vi "CSM-FileSyncWindow.vi"(7 "Name(FileSync)":string="FileSync") -> ()   [LabVIEW 2020, in "CSM-FileSync.lvlib"]
doc: "------------- lvcsm -------------\n[CSMStates]\nItem 0 = \"Event Structure\"\nItem 1 = \"Idle\"\nItem 2 = \"CSM Documentation\"\nItem 3 = \"VI Reference\"\nItem 4 = \"Error Handler\"\nItem 5 = \"Critical Error\"\nItem 6 = \"Target Timeout Error\"\nItem 7 = \"Target Error\"\nItem 8 = \"Async Response\"\nItem 9 = \"Response\"\nItem 10 = \"Async Message Posted\"\nItem 11 = \"Initialize Core Data\"\nItem 12 = \"Exit\"\nItem 13 = \"Data: Initialize\"\nItem 14 = \"Data: Cleanup\"\nItem 15 = \"Events: Register\"\nItem 16 = \"Events: Unregister\"\nItem 17 = \"UI: Initialize\"\nItem 18 = \"UI: Cursor Set\"\nItem 19 = \"UI: Front Panel State\"\nItem 20 = \"Macro: Initialize\"\nItem 21 = \"Macro: Exit\"\nItem 22 = \"API: Update List\"\nItem 23 = \"API: Update Connected Status\"\nItem 24 = \"API: Update Statusbar\"\nItem 25 = \"API: Link to Sync Engine\"\n\n[CSMStatus]\nItem 0 = \"Error Occurred@Error Handler\""
uses:
  CSM-FileSync.lvlib
  6641ad17-a0ad-4bac-bb5f-2ef3ab68202a.vi
  8cb7b144-fc6f-4ba1-ba8b-99306a1222b8.vi
  fb79005b-40a1-4b02-92b0-90b422e2c596.vi
  <userlib>/_NEVSTOP/Communicable State Machine(CSM)/AdvanceAPI/CSM - Revert Arguments-Safe String.vi
  <userlib>/_NEVSTOP/Communicable State Machine(CSM)/_Shared/Trim Single-line Text.vi
  <userlib>/_NEVSTOP/Communicable State Machine(CSM)/AdvanceAPI/CSM - Make String Arguments Safe.vi
  <userlib>/_NEVSTOP/Communicable State Machine(CSM)/AdvanceAPI/CSM - Break Down Multiple States String.vi
  <userlib>/_NEVSTOP/Communicable State Machine(CSM)/AdvanceAPI/CSM - Compact Multiple States.vi
  <userlib>/_NEVSTOP/Communicable State Machine(CSM)/AdvanceAPI/CSM - Keywords.vi
  <userlib>/_NEVSTOP/Communicable State Machine(CSM)/addons/MassData-Parameter/_support/FGV-MassData(lvlibp).vi
  <userlib>/_NEVSTOP/Communicable State Machine(CSM)/addons/API-String-Arugments-Support/_Support/Convert API String Arguments to Data(variant).vi
  <userlib>/_NEVSTOP/Communicable State Machine(CSM)/_Polymophic/CSM - Replace Marks in Messages.vi
  <userlib>/_NEVSTOP/Communicable State Machine(CSM)/Communicable State Machine.lvlib
panel:
  in  "Status":i32[](listbox)
  out "Statusbar":string
  out "Connected":bool
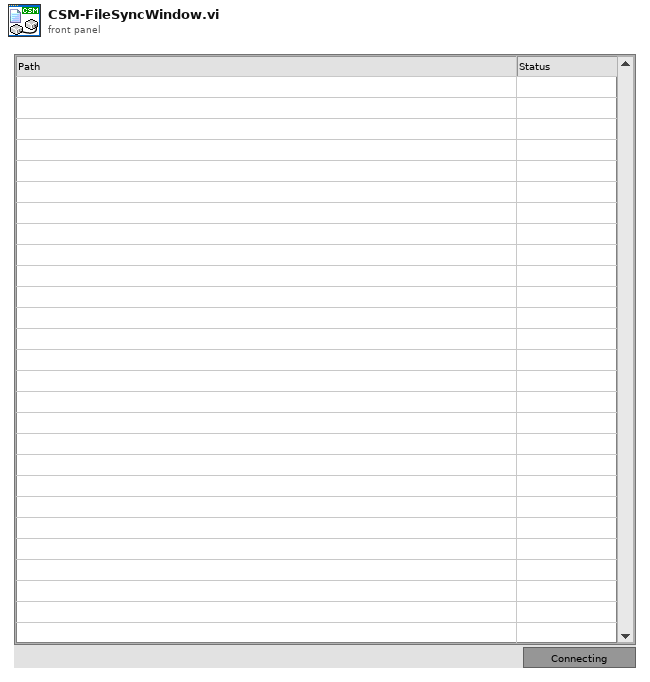
[diagram p1: front panel]
types:
  T1 = enum32{"Invalid", "Standard", "Closed", "Hidden", "Minimized", "Maximized"}
  T2 = enum32{"invalid app kind", "Development System", "Run Time System", "Student Edition", "Embedded LabVIEW", "Evaluation", "Custom"}
  T3 = cluster{"Upload List":path[], "UploadingFile":path}
  T4 = typedef "Communicable State Machine.lvlib/_CSM_Response Source Message.ctl" = cluster{"‘State":string, "’Arguments":string, "’Error":errorcluster}
  T5 = cluster{"Current VI Reference":refnum<vi>, "Close Panel on Exit?":bool}
  T6 = cluster{"Core":cluster{"Current VI Reference":refnum<vi>, "Close Panel on Exit?":bool}, "Status":refnum<vi>}
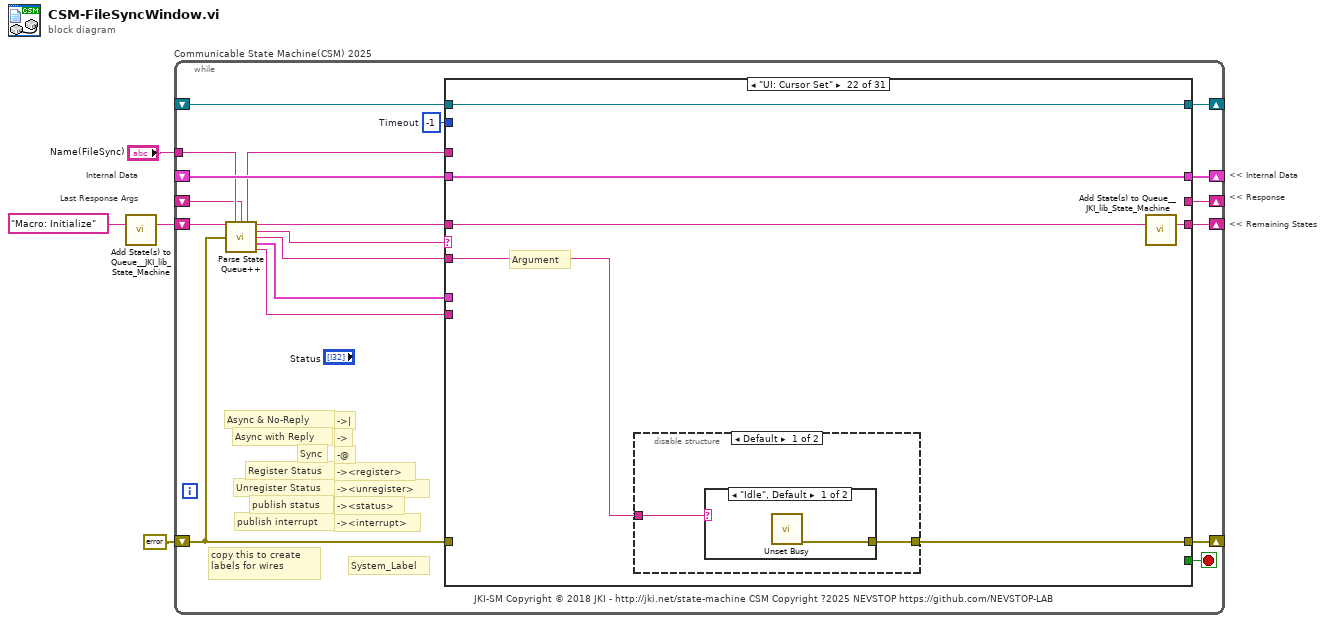
[diagram p0: block diagram]
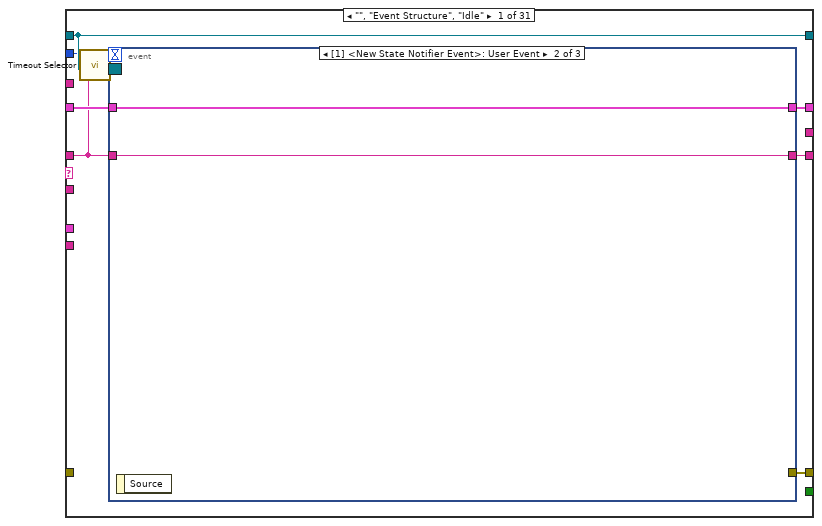
[diagram p2: hidden frame]
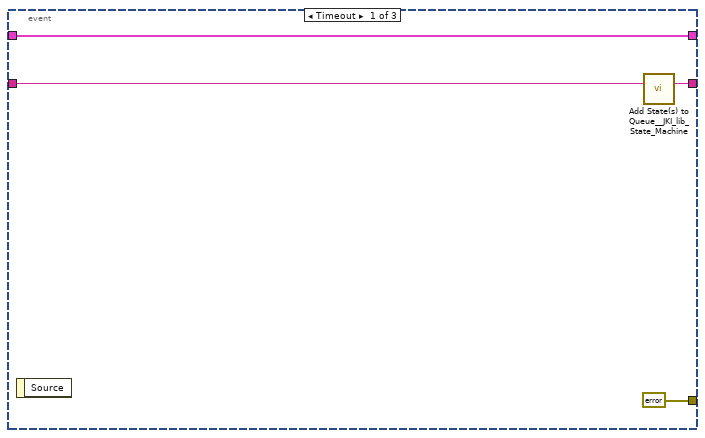
[diagram p3: hidden frame]
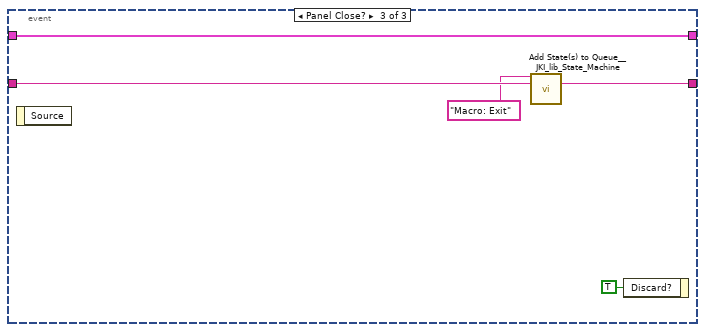
[diagram p4: hidden frame]
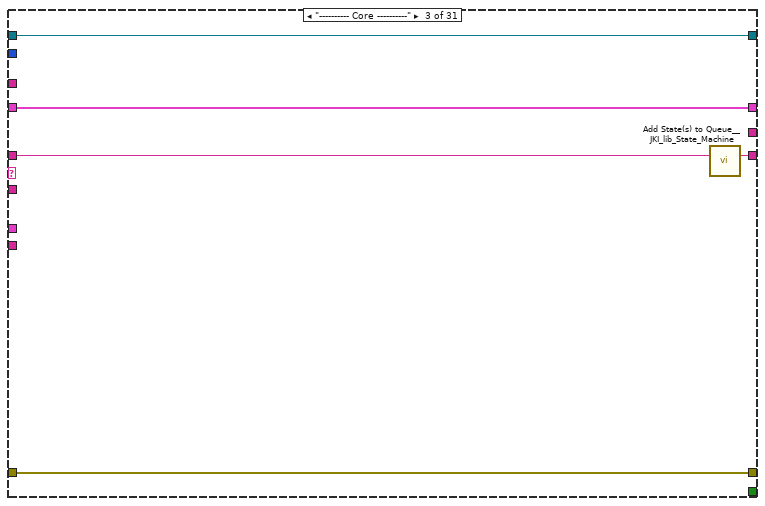
[diagram p6: hidden frame]
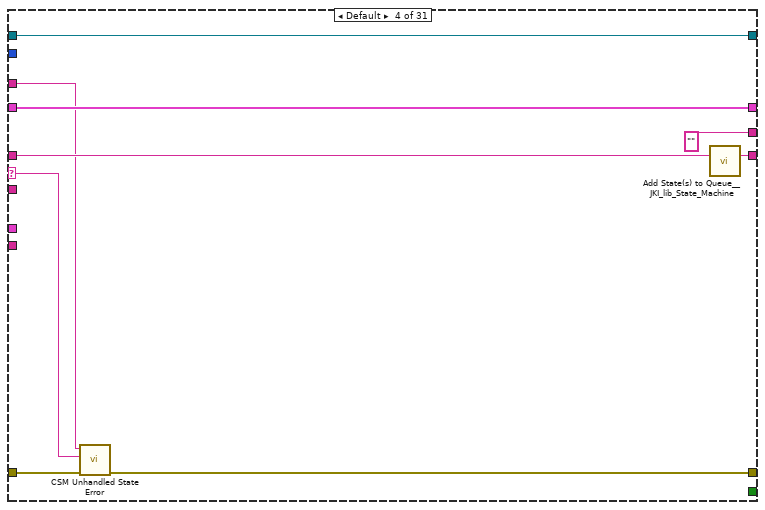
[diagram p7: hidden frame]
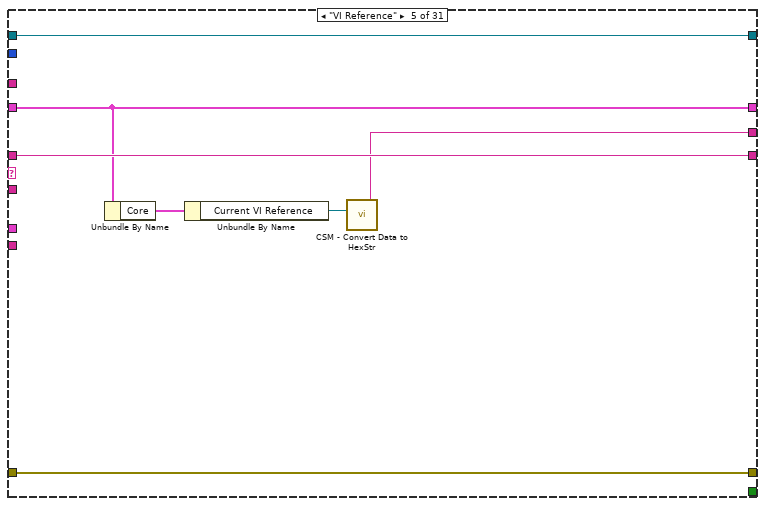
[diagram p8: hidden frame]
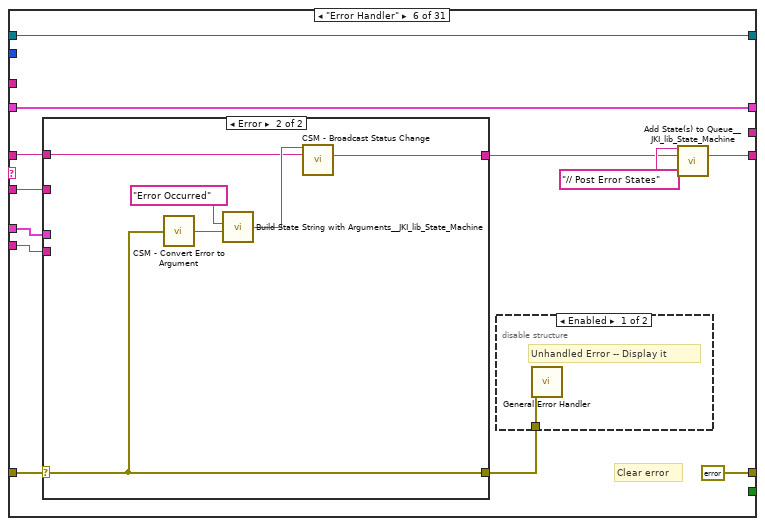
[diagram p9: hidden frame]
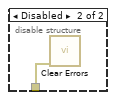
[diagram p10: hidden frame]
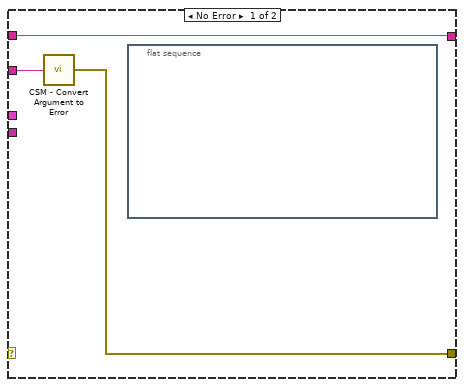
[diagram p11: hidden frame]
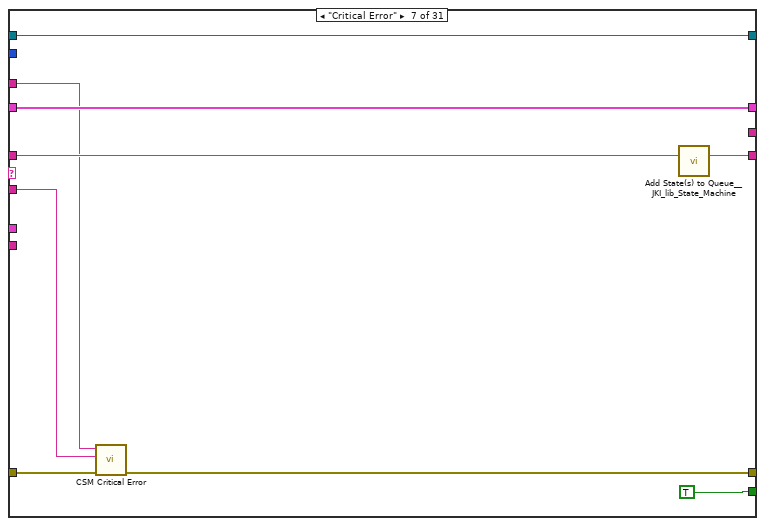
[diagram p12: hidden frame]
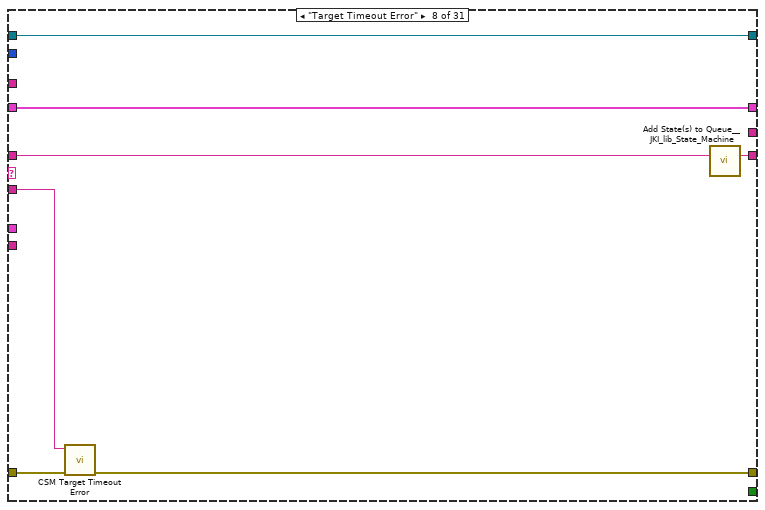
[diagram p13: hidden frame]
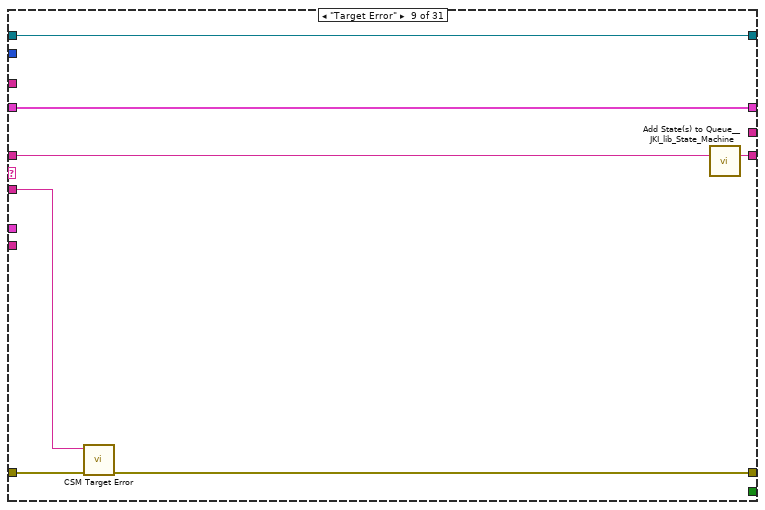
[diagram p14: hidden frame]
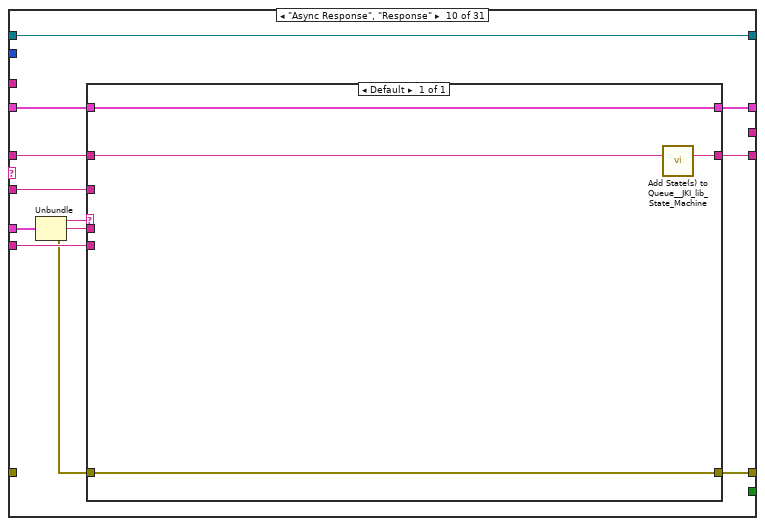
[diagram p15: hidden frame]
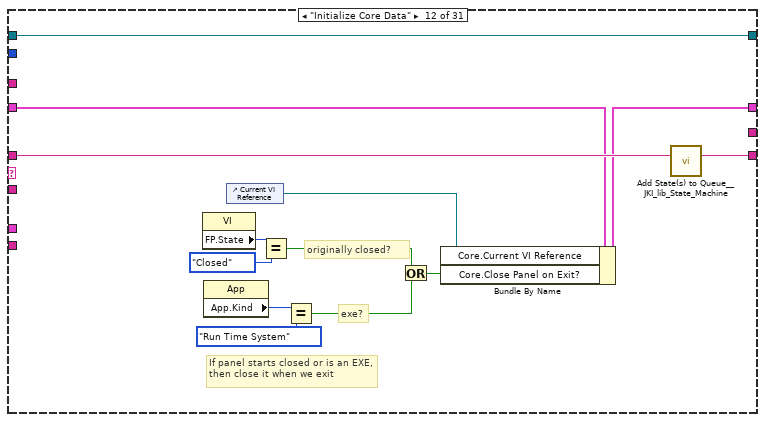
[diagram p17: hidden frame]
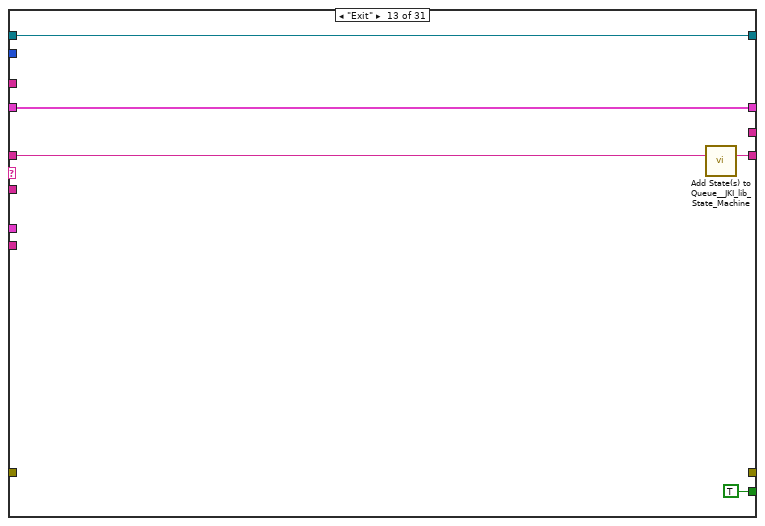
[diagram p18: hidden frame]
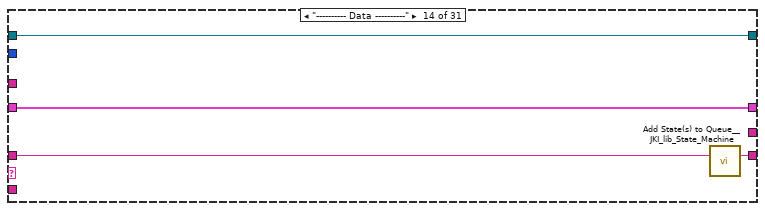
[diagram p19: hidden frame]
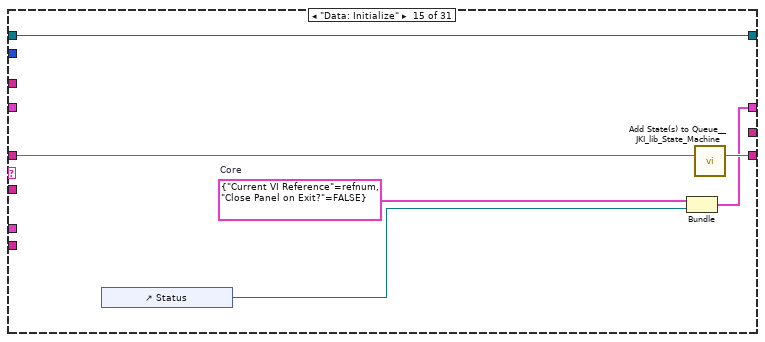
[diagram p20: hidden frame]
diagram:
  # "Last Response Args"
  # "Internal Data"
  # "<< Internal Data"
  # "<< Response"
  # "<< Remaining States"
  n1 = call <vilib>:"Add State(s) to Queue__JKI_lib_State_Machine.vi"("State(s) in (\"\")"="Macro: Initialize" ("Init State(\"Macro: Initialize\")")) -> ("States Out"=w3:string)  [unwired: 14 in]
  n2 = while "Communicable State Machine(CSM) 2025" {
    shift-right: [w18] -> _
    shift-left: _ -> [w17]
    shift-right: [w21] -> _
    shift-left: errorcluster {"status"=FALSE, "code"=0, "source"=""} ("error in") -> [w15]
    shift-right: [w20] -> _
    shift-left: w3 -> [w22]
    tunnel: "Name(FileSync)" -> [w11]
    shift-right: [w14] -> _
    shift-left: _ -> [w6]
    shift-right: [w13] -> _
    shift-left: _ -> [w12]
    stop <- w19 stop-if-true
    w16 = -1  # Timeout
    # "-><interrupt>"
    # "-><status>"
    # "-><unregister>"
    # "-><register>"
    # "-@"
    # "->"
    # "->|"
    # "publish interrupt"
    # "publish status"
    # "Unregister Status"
    # "Register Status"
    # "Sync"
    # "Async with Reply"
    # "Async & No-Reply"
    # "copy this to create labels for wires"
    # "System_Label"
    # "JKI-SM Copyright © 2018 JKI - http://jki.net/state-machine CSM Copyright ?2025 NEVSTOP https://github.com/NEVSTOP-LAB"
    n3 = call <userlib>:"Parse State Queue++.vi"("State Queue"=w22, "Name (\"\" to Use UUID)"=w11, "Response Arguments"=w6, "Previous Error"=w15) -> ("Name Used"=w7:string, "Remaining States"=w23:string, "Current State"=w10:string, "Arguments"=w5:string, "Additional Information"=w9:T4, "Source CSM"=w8:string)  [unwired: 6 in]
    n4 = case shown="\"UI: Cursor Set\"" w10 {
      selector: w10 -> [_ _ _ w53 _ _ _ _ _ _ _ _ _ _ _ _ _ _ _ _ _ _ _ _ _ _ _ _ _ _ _]
      tunnel: w23 -> [w24 w45 w50 w59 w65 w71 w97 w105 w112 w122 w131 w144 w149 w153 w159 w165 w169 w176 w180 w184 w188 w194 w205 w269 w274 w285 w288 w300 w311 w316 w323]
      tunnel: w5 -> [_ _ _ _ _ w69 w93 w100 w108 w116 _ _ _ _ _ _ _ _ _ _ _ w190 w200 _ _ _ _ w298 w306 w313 w320]
      tunnel: w17 -> [w30 w44 w47 w57 w64 w77 w98 w103 w110 w120 w130 w138 w147 w151 _ w161 w167 w175 w179 w182 w186 w192 w202 w267 w272 w283 w287 w297 w310 w315 w326]
      tunnel: [w29 _ w48 w51 w66 errorcluster {"status"=FALSE, "code"=0, "source"=""} ("error out") w90 w99 w106 w119 _ _ _ _ _ w162 _ w170 w178 _ _ w191 w203 _ _ _ _ w296 w312 w317 w327] -> w21
      tunnel: w15 -> [_ _ w48 w52 w66 w75 w91 w101 w107 _ _ _ _ _ _ _ _ _ _ _ _ _ _ _ _ _ _ _ w312 w317 w327]
      tunnel: [w31 w45 w49 w58 w65 w73 w96 w104 w111 w123 w131 w143 w148 w152 w158 w164 w168 w176 w180 w183 w187 w193 w204 w268 w273 w284 w288 w300 w311 w316 w324] -> w20
      tunnel: [_ _ _ _ _ _ TRUE _ _ _ _ _ TRUE _ _ _ _ _ _ _ _ _ _ _ _ _ _ _ _ _ _] -> w19
      tunnel: [w28 w44 w47 w57 w64 w77 w98 w103 w110 w121 w130 w142 w147 w151 w157 w161 w167 w175 w179 w182 w186 w192 w202 w267 w272 w283 w287 w297 w310 w315 w326] -> w18
      tunnel: w16 -> [w26 _ _ _ _ _ _ _ _ _ _ _ _ _ _ _ _ _ _ _ _ _ _ _ _ _ _ _ _ _ _]
      tunnel: w8 -> [_ _ _ _ _ w68 _ _ _ w117 _ _ _ _ _ _ _ _ _ _ _ _ _ _ _ _ _ _ _ _ _]
      tunnel: w9 -> [_ _ _ _ _ w67 _ _ _ w118 _ _ _ _ _ _ _ _ _ _ _ _ _ _ _ _ _ _ _ _ _]
      tunnel: [_ _ _ "" w60 _ _ _ _ _ _ _ _ _ _ _ _ _ _ _ _ _ _ _ _ _ _ _ _ _ _] -> w14
      tunnel: [w27 w43 w46 w55 w63 w76 w94 w102 w109 w124 w129 w132 w145 w150 w155 w160 w166 w174 w177 w181 w185 w189 w199 w266 w270 w276 w286 w299 w309 w314 w325] -> w13
      tunnel: w12 -> [w27 w43 w46 w55 w63 w76 w94 w102 w109 w124 w129 w132 w145 w150 w155 w160 w166 _ w177 w181 w185 w189 w199 w266 w270 w276 w286 w299 w309 w314 w325]
      tunnel: w7 -> [_ _ _ w54 _ _ w92 _ _ _ _ _ _ _ _ _ _ w173 _ _ _ _ _ _ _ _ _ _ _ _ _]
      frame "", "Event Structure", "Idle" {
        n5 = call <userlib>:"Timeout Selector.vi"("Remaining States"=w24, "Timeout Expected"=w26) -> ("Timeout"=w25:i32)  [unwired: 5 in]
        n6 = event shown="[1] <New State Notifier Event>: User Event" {
          selector: w27 -> [_ _ _]
          dyn-events: _ -> [_ _ _]
          timeout: w25 -> [_ _ _]
          tunnel: w24 -> [w35 w36 w42]
          tunnel: [w34 w36 w41] -> w31
          tunnel: w30 -> [w33 w37 w40]
          tunnel: [errorcluster {"status"=FALSE, "code"=0, "source"=""} ("error out") _ _] -> w29
          tunnel: [w33 w37 w40] -> w28
          event Timeout {
            n7 = event-data() -> ()  [unwired: 1 in, 1 out]
            n8 = call <vilib>:"Add State(s) to Queue__JKI_lib_State_Machine.vi"("State(s) in (\"\")"=w35) -> ("States Out"=w34:string)  [unwired: 14 in]
          }
          event User Event {
            n9 = event-data() -> ()  [unwired: 1 in, 1 out]
          }
          event Panel Close? {
            n10 = event-data() -> ()  [unwired: 1 in, 1 out]
            n11 = call <vilib>:"Add State(s) to Queue__JKI_lib_State_Machine.vi"("State(s) in Front (\"\")"="Macro: Exit", "State(s) in (\"\")"=w42) -> ("States Out"=w41:string)  [unwired: 13 in]
            n12 = event-data("Discard?"=TRUE) -> ()  [unwired: 1 in, 1 out]
          }
        }
      }
      frame "CSM Documentation" {
      }
      frame "---------- Core ----------" {
        n13 = call <vilib>:"Add State(s) to Queue__JKI_lib_State_Machine.vi"("State(s) in (\"\")"=w50) -> ("States Out"=w49:string)  [unwired: 14 in]
      }
      frame Default {
        n14 = call <userlib>:"CSM Unhandled State Error.vi"("error in (no error)"=w52, "Undefined State"=w53, "CSM Name"=w54) -> ("error out"=w51:errorcluster)  [unwired: 8 in]
        n15 = call <vilib>:"Add State(s) to Queue__JKI_lib_State_Machine.vi"("State(s) in (\"\")"=w59) -> ("States Out"=w58:string)  [unwired: 14 in]
      }
      frame "VI Reference" {
        n16 = Unbundle By Name(w64) -> ("Core"=w62:T5)
        n17 = Unbundle By Name(w62) -> ("Current VI Reference"=w61:refnum<vi>)
        n18 = call <userlib>:"CSM - Convert Data to HexStr.vi"("Variant"=w61) -> ("HEX String (0-9,A-F)"=w60:string)  [unwired: 8 in]
      }
      frame "Error Handler" {
        # "Clear error"
        n19 = case shown="Error" w75 {
          selector: w75 -> [_ w84]
          tunnel: [w82 w86] -> w72
          tunnel: w71 -> [w82 w85]
          tunnel: [w81 w84] -> w70
          tunnel: w69 -> [w83 _]
          tunnel: w68 -> [_ _]
          tunnel: w67 -> [_ _]
          frame No Error {
            n20 = call <userlib>:"CSM - Convert Argument to Error.vi"("Argument"=w83) -> ("Error"=w81:errorcluster)  [unwired: 4 in]
            n21 = flat-sequence {
              frame #0 {
              }
            }
          }
          frame Error {
            n22 = call <userlib>:"CSM - Convert Error to Argument.vi"("Error"=w84) -> ("Argument"=w88:string)  [unwired: 4 in]
            n23 = call <vilib>:"Build State String with Arguments__JKI_lib_State_Machine.vi"("Arguments (\"\")"=w88, "State"="Error Occurred" ("Status with Arguments")) -> ("State with Arguments"=w87:string)  [unwired: 4 in]
            n24 = call <userlib>:"CSM - Broadcast Status Change.vi"("Status With Arguments"=w87, "State Queue"=w85) -> ("Remaining States"=w86:string)  [unwired: 13 in]
          }
        }
        n25 = disable-structure shown="Enabled" {
          disable-tunnel: w70 -> [w79 w80]
          frame Enabled {
            # "Unhandled Error -- Display it"
            n26 = call <vilib>:"General Error Handler.vi"("error in (no error)"=w79) -> ()  [unwired: 10 in, 5 out]
          }
          frame Disabled {
            n27 = call <vilib>:"Clear Errors.vi"("error in (no error)"=w80) -> ()  [unwired: 5 in, 2 out]
          }
        }
        n28 = call <vilib>:"Add State(s) to Queue__JKI_lib_State_Machine.vi"("State(s) in Front (\"\")"="// Post Error States", "State(s) in (\"\")"=w72) -> ("States Out"=w73:string)  [unwired: 13 in]
      }
      frame "Critical Error" {
        n29 = call <userlib>:"CSM Critical Error.vi"("error in (no error)"=w91, "Arugments (As Reason)"=w93, "CSM Name"=w92) -> ("error out"=w90:errorcluster)  [unwired: 8 in]
        n30 = call <vilib>:"Add State(s) to Queue__JKI_lib_State_Machine.vi"("State(s) in (\"\")"=w97) -> ("States Out"=w96:string)  [unwired: 14 in]
      }
      frame "Target Timeout Error" {
        n31 = call <userlib>:"CSM Target Timeout Error.vi"("error in (no error)"=w101, "Arguments (As CSM Name)"=w100) -> ("error out"=w99:errorcluster)  [unwired: 9 in]
        n32 = call <vilib>:"Add State(s) to Queue__JKI_lib_State_Machine.vi"("State(s) in (\"\")"=w105) -> ("States Out"=w104:string)  [unwired: 14 in]
      }
      frame "Target Error" {
        n33 = call <userlib>:"CSM Target Error.vi"("error in (no error)"=w107, "Arguments (As CSM Name)"=w108) -> ("error out"=w106:errorcluster)  [unwired: 9 in]
        n34 = call <vilib>:"Add State(s) to Queue__JKI_lib_State_Machine.vi"("State(s) in (\"\")"=w112) -> ("States Out"=w111:string)  [unwired: 14 in]
      }
      frame "Async Response", "Response" {
        n35 = Unbundle(w118) -> ("‘State"=w115:string, "’Arguments"=w114:string, "’Error"=w113:errorcluster)
        n36 = case shown="Default" w115 {
          tunnel: [w125] -> w123
          tunnel: w122 -> [w126]
          tunnel: [w128] -> w121
          tunnel: w120 -> [w128]
          tunnel: [w127] -> w119
          tunnel: w113 -> [w127]
          tunnel: w117 -> [_]
          tunnel: w116 -> [_]
          tunnel: w114 -> [_]
          frame Default {
            n37 = call <vilib>:"Add State(s) to Queue__JKI_lib_State_Machine.vi"("State(s) in (\"\")"=w126) -> ("States Out"=w125:string)  [unwired: 14 in]
          }
        }
      }
      frame "Async Message Posted" {
      }
      frame "Initialize Core Data" {
        # "originally closed?"
        # "exe?"
        # "If panel starts closed or is an EXE, then close it when we exit"
        n38 = property class="VI"() -> ("FP.State"=w135:T1)  [unwired: 2 in, 2 out]
        n39 = property class="App"() -> ("App.Kind"=w141:T2)  [unwired: 2 in, 2 out]
        n40 = control-ref of="Current VI Reference"() -> (w136:refnum<vi>)
        n41 = Equal?(x=w135, y=T1."Closed" ("Front Panel Window:State")) -> (x = y?=w133:bool)
        n42 = Equal?(x=w141, y=T2."Run Time System" ("Application:Kind")) -> (x = y?=w139:bool)
        n43 = Or(x=w133, y=w139) -> (x .or. y?=w137:bool)
        n44 = Bundle By Name(cluster=w138, "Core.Current VI Reference"=w136, "Core.Close Panel on Exit?"=w137) -> (w142:T6)
        n45 = call <vilib>:"Add State(s) to Queue__JKI_lib_State_Machine.vi"("State(s) in (\"\")"=w144) -> ("States Out"=w143:string)  [unwired: 14 in]
      }
      frame "Exit" {
        n46 = call <vilib>:"Add State(s) to Queue__JKI_lib_State_Machine.vi"("State(s) in (\"\")"=w149) -> ("States Out"=w148:string)  [unwired: 14 in]
      }
      frame "---------- Data ----------" {
        n47 = call <vilib>:"Add State(s) to Queue__JKI_lib_State_Machine.vi"("State(s) in (\"\")"=w153) -> ("States Out"=w152:string)  [unwired: 14 in]
      }
      frame "Data: Initialize" {
        w156 = T5 {"Current VI Reference"=refnum, "Close Panel on Exit?"=FALSE}  # Core
        n48 = control-ref of="Status"() -> (w154:refnum<vi>)
        n49 = Bundle("Core"=w156, "Status"=w154) -> (w157:T6)  [unwired: 1 in]
        n50 = call <vilib>:"Add State(s) to Queue__JKI_lib_State_Machine.vi"("State(s) in (\"\")"=w159) -> ("States Out"=w158:string)  [unwired: 14 in]
      }
      frame "Data: Cleanup" {
        n51 = Unbundle By Name(w161) -> ("Core.Current VI Reference"=w163:refnum<vi>)
        n52 = Close Reference(reference=w163) -> (error out=w162:errorcluster)  [unwired: 1 in]
        n53 = call <vilib>:"Add State(s) to Queue__JKI_lib_State_Machine.vi"("State(s) in (\"\")"=w165) -> ("States Out"=w164:string)  [unwired: 14 in]
      }
      frame "---------- Events ----------" {
        n54 = call <vilib>:"Add State(s) to Queue__JKI_lib_State_Machine.vi"("State(s) in (\"\")"=w169) -> ("States Out"=w168:string)  [unwired: 14 in]
      }
      frame "Events: Register" {
        n55 = call <userlib>:"CSM - Get New State Notifier Event.vi"("Name (\"\" to Use UUID)"=w173) -> ("error out"=w171:errorcluster, "New State Notifier Event"=w172:refnum<user-event>)  [unwired: 9 in]
        n56 = register-events(error in=w171, w172) -> (reference out=w174:refnum<event-registration>, error out=w170:errorcluster)  [unwired: 1 in]
      }
      frame "Events: Unregister" {
        n57 = Unregister For Events(event registration refnum=w177) -> (error out=w178:errorcluster)  [unwired: 1 in]
      }
      frame "---------- UI ----------" {
        n58 = call <vilib>:"Add State(s) to Queue__JKI_lib_State_Machine.vi"("State(s) in (\"\")"=w184) -> ("States Out"=w183:string)  [unwired: 14 in]
      }
      frame "UI: Initialize" {
        n59 = call <vilib>:"Add State(s) to Queue__JKI_lib_State_Machine.vi"("State(s) in (\"\")"=w188) -> ("States Out"=w187:string)  [unwired: 14 in]
      }
      frame "UI: Cursor Set" {
        # "Argument"
        n60 = disable-structure shown="Default" {
          disable-tunnel: [w196 _] -> w191
          disable-tunnel: w190 -> [w195 _]
          frame condition #0 (active) {
            n61 = case shown="\"Idle\", Default" w195 {
              tunnel: [w197 w198] -> w196
              frame "Idle", Default {
                n62 = call <vilib>:"Unset Busy.vi"() -> ("error out"=w197:errorcluster)  [unwired: 11 in]
              }
              frame "Busy" {
                n63 = call <vilib>:"Set Busy.vi"() -> ("error out"=w198:errorcluster)  [unwired: 10 in, 1 out]
              }
            }
          }
          frame condition #1 {
          }
        }
        n64 = call <vilib>:"Add State(s) to Queue__JKI_lib_State_Machine.vi"("State(s) in (\"\")"=w194) -> ("States Out"=w193:string)  [unwired: 14 in]
      }
      frame "UI: Front Panel State" {
        # "Argument"
        n65 = Unbundle By Name(w202) -> ("Core.Current VI Reference"=w201:refnum<vi>)
        n66 = case shown="\"Minimize\", \"Minimized\"" w200 {
          tunnel: [w212 w225 w236 w248 w260] -> w203
          tunnel: w201 -> [w211 w223 w235 w247 w259]
          frame "Open", "Standard", Default {
            w206 = T1."Standard" ("State")
            n67 = property class="VI"(reference=w211) -> (reference out=w209:refnum<vi>, error out=w210:errorcluster, "FP.State"=w208:T1)  [unwired: 1 in]
            n68 = Not Equal?(x=w208, y=w206) -> (x != y?=w207:bool)
            n69 = case shown="True" w207 {
              tunnel: [w216 w218] -> w212
              tunnel: w210 -> [w215 w218]
              tunnel: w209 -> [w214 _]
              tunnel: w206 -> [w213 _]
              frame True {
                n70 = invoke class="VI" method="FP.Open"(reference=w214, error in=w215, "Activate"=TRUE, "State"=w213) -> (error out=w216:errorcluster)  [unwired: 1 in, 4 out]
              }
              frame False {
              }
            }
          }
          frame "Close", "Closed" {
            n71 = property class="VI"(reference=w223) -> (reference out=w222:refnum<vi>, error out=w224:errorcluster, "FP.State"=w220:T1)  [unwired: 1 in]
            n72 = Not Equal?(x=w220, y=T1."Closed" ("Front Panel Window:State")) -> (x != y?=w219:bool)
            n73 = case shown="True" w219 {
              tunnel: [w226 w229] -> w225
              tunnel: w224 -> [w226 w228]
              tunnel: w222 -> [_ w227]
              frame False {
              }
              frame True {
                n74 = invoke class="VI" method="FP.Close"(reference=w227, error in=w228) -> (error out=w229:errorcluster)  [unwired: 1 in, 2 out]
              }
            }
          }
          frame "Hidden", "Hide" {
            w230 = T1."Hidden" ("State")
            n75 = property class="VI"(reference=w235) -> (reference out=w233:refnum<vi>, error out=w234:errorcluster, "FP.State"=w232:T1)  [unwired: 1 in]
            n76 = Not Equal?(x=w232, y=w230) -> (x != y?=w231:bool)
            n77 = case shown="True" w231 {
              tunnel: [w240 w241] -> w236
              tunnel: w234 -> [w239 w241]
              tunnel: w233 -> [w238 _]
              tunnel: w230 -> [w237 _]
              frame True {
                n78 = invoke class="VI" method="FP.Open"(reference=w238, error in=w239, "State"=w237) -> (error out=w240:errorcluster)  [unwired: 2 in, 4 out]
              }
              frame False {
              }
            }
          }
          frame "Minimize", "Minimized" {
            w242 = T1."Minimized" ("State")
            n79 = property class="VI"(reference=w247) -> (reference out=w245:refnum<vi>, error out=w246:errorcluster, "FP.State"=w244:T1)  [unwired: 1 in]
            n80 = Not Equal?(x=w244, y=w242) -> (x != y?=w243:bool)
            n81 = case shown="False" w243 {
              tunnel: [w252 w253] -> w248
              tunnel: w246 -> [w251 w253]
              tunnel: w245 -> [w250 _]
              tunnel: w242 -> [w249 _]
              frame True {
                n82 = invoke class="VI" method="FP.Open"(reference=w250, error in=w251, "State"=w249) -> (error out=w252:errorcluster)  [unwired: 2 in, 4 out]
              }
              frame False {
              }
            }
          }
          frame "Maximize", "Maximized" {
            w254 = T1."Maximized" ("State")
            n83 = property class="VI"(reference=w259) -> (reference out=w257:refnum<vi>, error out=w258:errorcluster, "FP.State"=w256:T1)  [unwired: 1 in]
            n84 = Not Equal?(x=w256, y=w254) -> (x != y?=w255:bool)
            n85 = case shown="True" w255 {
              tunnel: [w264 w265] -> w260
              tunnel: w258 -> [w263 w265]
              tunnel: w257 -> [w262 _]
              tunnel: w254 -> [w261 _]
              frame True {
                n86 = invoke class="VI" method="FP.Open"(reference=w262, error in=w263, "State"=w261) -> (error out=w264:errorcluster)  [unwired: 2 in, 4 out]
              }
              frame False {
              }
            }
          }
        }
        n87 = call <vilib>:"Add State(s) to Queue__JKI_lib_State_Machine.vi"("State(s) in (\"\")"=w205) -> ("States Out"=w204:string)  [unwired: 14 in]
      }
      frame "---------- Macro ----------" {
        n88 = call <vilib>:"Add State(s) to Queue__JKI_lib_State_Machine.vi"("State(s) in (\"\")"=w269) -> ("States Out"=w268:string)  [unwired: 14 in]
      }
      frame "Macro: Initialize" {
        w271 = "Data: Initialize\nInitialize Core Data\nEvents: Register\nUI: Initialize\n//UI: Front Panel State >> Open"  # Data: Initialize Initialize Core Data Events: Register UI: Initialize //UI: Front Panel State >> Open
        n89 = call <vilib>:"Add State(s) to Queue__JKI_lib_State_Machine.vi"("State(s) in Front (\"\")"=w271, "State(s) in (\"\")"=w274) -> ("States Out"=w273:string)  [unwired: 13 in]
      }
      frame "Macro: Exit" {
        n90 = Unbundle By Name(w283) -> ("Core.Close Panel on Exit?"=w282:bool)
        n91 = Select(t="UI: Front Panel State >> Close", s=w282, f="") -> (s? t:f=w279:string)
        n92 = call <vilib>:"Add State(s) to Queue__JKI_lib_State_Machine.vi"("State(s) in Front (\"\")"="//Exit Sub-Modules ", "State(s) in (\"\")"=w279, "State(s) at Back (\"\")"="Data: Cleanup\nEvents: Unregister\nExit") -> ("States Out"=w277:string)  [unwired: 12 in]
        n93 = call <vilib>:"Add State(s) to Queue__JKI_lib_State_Machine.vi"("State(s) in Front (\"\")"=w277, "State(s) in (\"\")"=w285) -> ("States Out"=w284:string)  [unwired: 13 in]
      }
      frame "---------- API ----------" {
      }
      frame "API: Update List" {
        n94 = Unbundle By Name(w297) -> ("Status"=w294:refnum<vi>)
        n95 = call "CSM - Convert Argument to MassData.vim"("Type"=T3 {"Upload List"=[], "UploadingFile"=path ""} ("output cluster"), "MassData Argument"=w298) -> ("error out"=w296:errorcluster, "Data"=w293:T3)  [unwired: 6 in]
        n96 = feedback-in #1(w293) -> ()
        n97 = feedback #1() -> (w292:T3)  [unwired: 1 in]
        n98 = Not Equal?(x=w293, y=w292) -> (x != y?=w290:bool)
        n99 = First Call?() -> (First Call?: T/F=w289:bool)
        n100 = Or(x=w290, y=w289) -> (x .or. y?=w291:bool)
        n101 = case shown="True" w291 {
          tunnel: w294 -> [_ w303]
          tunnel: w293 -> [_ w302]
          frame False {
          }
          frame True {
            n102 = Unbundle(w302) -> ("Upload List"=w305:path[], "UploadingFile"=w304:path)
            n103 = call "Prepare Status Table.vi"("MulticolumnListbox in"=w303, "Temp:UploadingFile"=w304, "Upload List"=w305) -> ("Array"=w301:string[][])  [unwired: 8 in]
            n104 = property class="MCListbox (strict)"(reference=w303, "ItemNames"=w301) -> ()  [unwired: 1 in, 2 out]
          }
        }
      }
      frame "API: Update Connected Status" {
        n105 = call "Convert API String Arguments to Data.vim"("Reference Type"=FALSE, "API String"=w306) -> ("Data"=→"Connected":bool)  [unwired: 6 in, 1 out]
      }
      frame "API: Update Statusbar" {
        "Statusbar" <- w313
      }
      frame "API: Link to Sync Engine" {
        n106 = call "Convert API String Arguments to Data.vim"("Reference Type"="FileSync" ("Name(FileSync)"), "API String"=w320) -> ("Data"=w318:string)  [unwired: 6 in, 1 out]
        n107 = call-poly <userlib>:"Build Message with Arguments++.vi"("States With Replace Token"="Status Change@<1> >> API: Update Connected Status -><register> \nUploading List Change@<1> >> API: Update List -><register> " ("State(s) in Front (\"\")"), "<1>"=w318) -> ("States"=w321:string)  [unwired: 13 in]
        n108 = call <vilib>:"Add State(s) to Queue__JKI_lib_State_Machine.vi"("State(s) in Front (\"\")"=w321, "State(s) in (\"\")"=w323) -> ("States Out"=w324:string)  [unwired: 13 in]
      }
    }
  }
